vi "GetText.vi"(8 "error in":errorcluster, 11 "node in":refnum<class "Targets.lvclass">) -> (0 "error out":errorcluster, 1 "additional text":string, 2 "text":string, 3 "node out":refnum<class "Targets.lvclass">, 4 "glyph":string)   [LabVIEW 2013, in "PL Framework Configuration Tool.lvlib" / "Targets.lvclass"]
doc: "Returns the text representation of the node used for the tree control."
uses:
  Targets.lvclass
  subVIs/Glyphs Status.ctl
  Framework Configuration Classes/target configuration/PL_Target Configuration.lvclass
  Framework Configuration Classes/target configuration/PL_Target Configuration.lvclass/PL_Target Configuration.ctl
  PL Framework Configuration Tool.lvlib
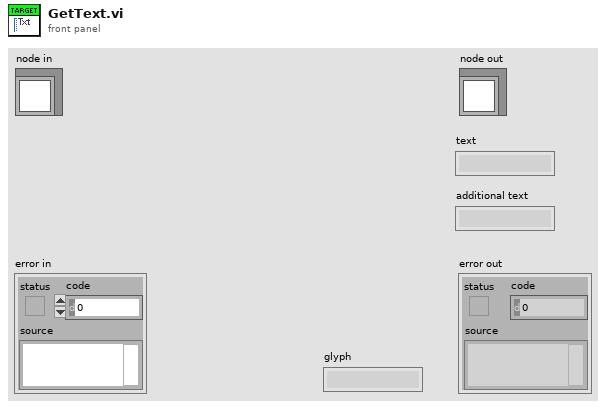
[diagram p1: front panel]
types:
  T1 = typedef "PL Framework Configuration Tool.lvlib/Glyphs Status.ctl" = enum16{"Normal", "Error", "Async"}
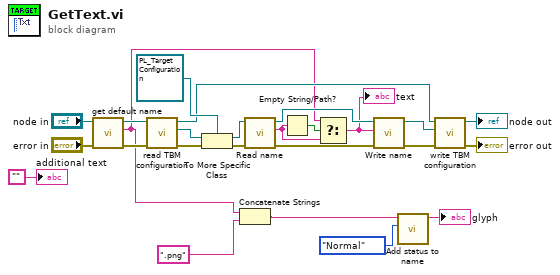
[diagram p0: block diagram]
diagram:
  n1 = call-dynamic "get default name.vi"("error in"="error in", "Targets in"="node in") -> ("error out"=w15:errorcluster, "default name"=w3:string, "Targets out"=w16:refnum<class "Targets.lvclass">)  [unwired: 7 in]
  n2 = call-dynamic "read TBM configuration.vi"("error in"=w15, "TBM Configuration Node in"=w16) -> ("error out"=w12:errorcluster, "configuration"=w14:refnum<class "TBM configuration.lvclass">, "TBM Configuration Node out"=w13:refnum<class "Targets.lvclass">)  [unwired: 7 in]
  n3 = To More Specific Class(target class=refnum<class "PL_Target Configuration.lvclass"> refnum ("Target Configuration"), reference=w14, error in=w12) -> (specific class reference=w10:refnum<class "PL_Target Configuration.lvclass">, error out=w11:errorcluster)
  n4 = Concatenate Strings(w3, ".png" ("glyph")) -> (w1:string)
  n5 = call "Read name.vi"("error in"=w11, "PL_Local Target Configuration in"=w10) -> ("error out"=w7:errorcluster, "name"=w9:string, "PL_Local Target Configuration out"=w8:refnum<class "PL_Target Configuration.lvclass">)  [unwired: 7 in]
  n6 = Empty String/Path?(string/path=w9) -> (empty?=w21:bool)
  n7 = Select(t=w3, s=w21, f=w9) -> (s? t:f=w6:string)
  "text" <- w6
  n8 = call "Write name.vi"("error in"=w7, "name"=w6, "PL_Local Target Configuration in"=w8) -> ("error out"=w5:errorcluster, "PL_Local Target Configuration out"=w4:refnum<class "PL_Target Configuration.lvclass">)  [unwired: 7 in]
  n9 = call "Add status to name.vi"("Status"=Glyphs_Status."Normal", "Name"=w1) -> ("Name with status"=→"glyph":string)  [unwired: 9 in]
  n10 = call-dynamic "write TBM configuration.vi"("error in"=w5, "configuration"=w4, "TBM Configuration Node in"=w13) -> ("error out"=→"error out":errorcluster, "TBM Configuration Node out"=→"node out":refnum<class "Targets.lvclass">)  [unwired: 7 in]
  "additional text" <- ""
